vi "View-grabber-settings-with-dialog.vi"(8 "error in (no error)":errorcluster, 10 "UI ref. in":refnum<data-value>, 11 "Data ref. in":refnum<data-value>) -> (0 "error out":errorcluster, 3 "Data ref.":refnum<data-value>)   [LabVIEW 2013, in "CameraVision.lvlib" / "CV-Main.lvclass"]
uses:
  CV-Main.lvclass
  UI/CV-UI.lvclass
  CV-Main.lvclass/CV-Main.ctl
  Storage/CV-Storage.lvclass/CV-Storage.ctl
  UI/CV-UI.lvclass/CV-UI.ctl
  Configuration/CV-Configuration.lvclass/CV-Configuration.ctl
  UI/Read Camera.vi
  Read Config params.vi
  Read Storage params.vi
  Storage/Read Base path.vi
  Configuration/Read Framegrabber DLL file.vi
  Configuration/Read Framegrabber board.vi
  Configuration/Read Camport array.vi
  Configuration/Read Camera config file.vi
  Configuration/CV-Configuration.lvclass
  Storage/CV-Storage.lvclass
panel:
  out "Ready":bool
  in  "OK":bool
  out "Grabber settings":cluster{"Name":string, "Value":i32}[](array[cluster])
  in  "Get parameter":i32(ring)=200 items=["FG_WIDTH"=100, "FG_HEIGHT"=200, "FG_FORMAT"=700, "FG_XOFFSET"=300, "FG_YOFFSET"=400, "FG_FRAMESPERSEC"=90, "FG_EXPOSURE"=10020, "FG_TRIGGERMODE"=8100, "FG_TRIGGERINSRC"=8110, "FG_CAMERA_LINK_CAMTYP"=11011, "FG_USEDVAL"=5025, "FG_SENSORREADOUT"=5050, "FG_STROBEPULSEDELAY"=8700, "FG_FLASH_POLARITY"=24060, "FG_EXSYNCINVERT"=8200, "FG_EXSYNCPOLARITY"=8420, "FG_EXSYNCDELAY"=8400, "FG_FLASHON"=8600, "FG_EXSYNCON"=8300, "FG_TRIGGERINPOLARITY"=8116, "FG_KNEE_LUT_FILE"=12110, "FG_KNEE_LUT_OFFSET"=12102, "FG_KNEE_LUT_SCALE"=12101, "FG_KNEE_LUT_GAMMA"=12103, "FG_KNEE_LUT_INVERT"=12104, "FG_CCSEL0"=14001, "FG_CCSEL1"=14002, "FG_CCSEL2"=14003, "FG_CCSEL3"=14004, "FG_DIGIO_OUTPUT"=14020, "FG_IMG_SELECT_PERIOD"=25110, "FG_IMG_SELECT"=25111, "FG_PORT"=3000, "FG_GLOBAL_ACCESS"=24110, "FG_TIMEOUT"=600]
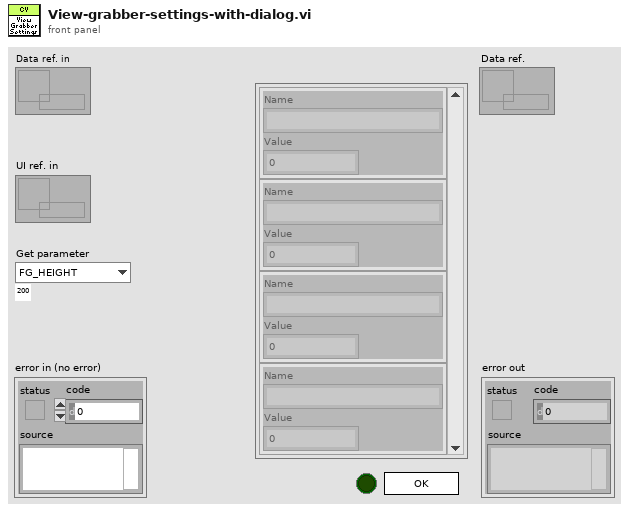
[diagram p1: front panel]
types:
  T1 = typedef "LVStringsAndValuesArrayTypeDef_I32.ctl" = cluster{"String":string, "Value":i32}[]
  T2 = typedef "CameraVision.lvlib/CV-UI.lvclass/Camera-selector.ctl" = enum16{"Camera 1", "Camera 2"}
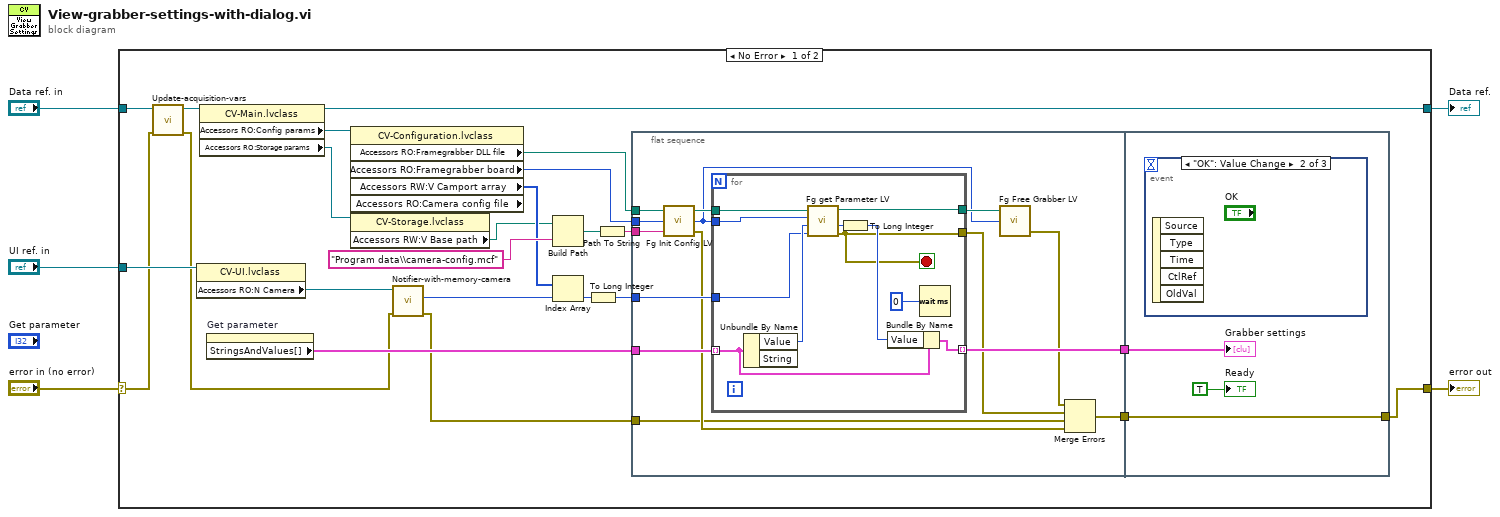
[diagram p0: block diagram]
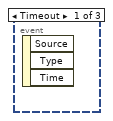
[diagram p2: hidden frame]
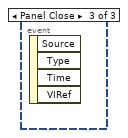
[diagram p3: hidden frame]
diagram:
  n1 = case shown="No Error" "error in (no error)" {
    selector: "error in (no error)" -> [w9 w59]
    tunnel: [w16 w59] -> w4
    tunnel: [w29 w58] -> w2
    tunnel: "Data ref. in" -> [w11 w58]
    tunnel: "UI ref. in" -> [w21 _]
    frame No Error {
      n2 = call "Update-acquisition-vars.vi"("error in"=w9, "Data ref. in"=w11) -> ("error IO"=w8:errorcluster, "Data ref."=w10:refnum<data-value>)  [unwired: 6 in, 2 out]
      n3 = property class="CV-UI.lvclass"(reference=w21) -> ("Accessors RO:N Camera"=w15:refnum<notifier>)  [unwired: 1 in, 2 out]
      n4 = property class="CV-Main.lvclass"(reference=w10) -> (reference out=w29:refnum<data-value>, "Accessors RO:Config params"=w28:refnum<data-value>, "Accessors RO:Storage params"=w7:refnum<data-value>)  [unwired: 1 in, 1 out]
      n5 = property on="Get parameter" class="Ring (strict)"() -> ("StringsAndValues[]"=w22:T1)  [unwired: 2 in, 2 out]
      n6 = property class="CV-Configuration.lvclass" props=["Accessors RO:Framegrabber DLL file", "Accessors RO:Framegrabber board", "Accessors RW:V Camport array", "Accessors RO:Camera config file"](reference=w28) -> ("Accessors RO:Framegrabber DLL file"=w27:path, "Accessors RO:Framegrabber board"=w23:i32, "Accessors RW:V Camport array"=w13:u32[])  [unwired: 1 in, 3 out]
      n7 = property class="CV-Storage.lvclass"(reference=w7) -> ("Accessors RW:V Base path"=w6:path)  [unwired: 1 in, 2 out]
      n8 = call "Notifier-with-memory-camera.vi"("error in"=w8, "Notifier in"=w15) -> ("error IO"=w14:errorcluster, "Notification"=w12:T2)  [unwired: 8 in]
      n9 = Build Path(base path=w6, name or relative path="Program data\\camera-config.mcf") -> (appended path=w24:path)
      n10 = Index Array(array=w13, index=w12) -> (element=w20:u32)
      n11 = To Long Integer(number=w20) -> (32bit integer=w19:i32)
      n12 = Path To String(path=w24) -> (string=w25:string)
      n13 = flat-sequence {
        tunnel: w27 -> [w43]
        tunnel: w25 -> [w42]
        tunnel: w23 -> [w41]
        tunnel: w22 -> [w39]
        tunnel: w19 -> [w38]
        tunnel: w14 -> [w31]
        tunnel: [w37] -> w18
        tunnel: [w30] -> w17
        tunnel: w18 -> [w57]
        tunnel: w17 -> [w55]
        tunnel: [w55] -> w16
        frame #0 {
          n14 = call <userlib>:"Fg Init Config LV.vi"("Config_Name"=w42, "NumberOfmEnable"=w41, "dll path in"=w43) -> ("error out"=w32:errorcluster, "function return"=w35:u64, "dll path out"=w40:path)
          n15 = for {
            tunnel: w40 -> [w54]
            tunnel: w39 -> [w48] mode=indexing
            tunnel: w35 -> [w51]
            tunnel: w38 -> [w50]
            tunnel: [w47] -> w37 mode=indexing
            tunnel: [w45] -> w36
            tunnel: [w44] -> w33
            stop <- w44 stop-if-true
            n16 = Unbundle By Name(w48) -> ("Value"=w52:i32)  [unwired: 1 out]
            n17 = call <userlib>:"Fg get Parameter LV.vi"("CamPort"=w50, "Parameter"=w52, "FgAddr"=w51, "dll path in"=w54) -> ("error out"=w44:errorcluster, "Value out"=w49:u32, "dll path out"=w45:path)  [unwired: 1 out]
            n18 = To Long Integer(number=w49) -> (32bit integer=w46:i32)
            n19 = Bundle By Name(cluster=w48, "Value"=w46) -> (w47:cluster{"String":string, "Value":i32})
            n20 = Wait (ms)(milliseconds to wait=u32 0) -> ()  [unwired: 1 out]
          }
          n21 = call <userlib>:"Fg Free Grabber LV.vi"("FgAddr"=w35, "dll path in"=w36) -> ("error out"=w34:errorcluster)  [unwired: 1 in, 2 out]
          n22 = Merge Errors(w34, w33, w31, w32) -> (w30:errorcluster)
        }
        frame #1 {
          n23 = event shown="[1] \"OK\": Value Change" {
            selector: _ -> [_ _ _]
            dyn-events: _ -> [_ _ _]
            timeout: _ -> [_ _ _]
            event Timeout {
              n24 = event-data() -> ()  [unwired: 1 in, 3 out]
            }
            event "OK": Value Change {
              n25 = event-data() -> ()  [unwired: 1 in, 5 out]
            }
            event Panel Close {
              n26 = event-data() -> ()  [unwired: 1 in, 4 out]
            }
          }
          "Grabber settings" <- w57
          "Ready" <- TRUE ("Ready")
        }
      }
    }
    frame Error {
    }
  }
  "error out" <- w4
  "Data ref." <- w2
